vi "DrawArrowedLineOnImageARGB.vi"(4 "Thickness (Default: 1)":i32=1, 5 "Tip Length (Default 0.1)":dbl=0.1, 6 "ARGB Colour":T2={"Alpha"=255, "RGB"=0}, 7 "OpenCV Line Type (Default LINE_8)":T3=enum."LINE_8", 8 "error in (no error)":errorcluster, 9 "Pointed-to Point":T1, 10 "Start Point":T1, 11 "ARGB Image":refnum<data-value>) -> (0 "error out":errorcluster, 3 "ARGB Image (Duplicate)":refnum<data-value>)   [LabVIEW 2020, in "g_ar_toolkit.image.lvlib"]
uses:
  g_ar_toolkit.image.lvlib
  Line Type.ctl
  Image Point (Fixed).ctl
  ARGB Colour.ctl
  <vilib>/Utility/error.llb/Error Cluster From Error Code.vi
  c990ea83-8feb-41a3-987e-5529af170d73.vi
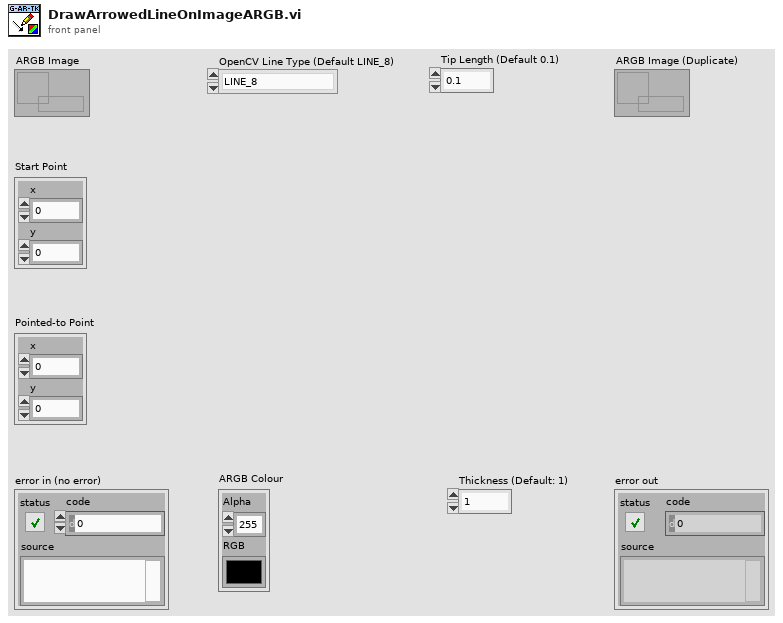
[diagram p1: front panel]
types:
  T1 = typedef "g_ar_toolkit.image.lvlib/Image Point (Fixed).ctl" = cluster{"x":i32, "y":i32}
  T2 = typedef "g_ar_toolkit.image.lvlib/ARGB Colour.ctl" = cluster{"Alpha":u8, "RGB":u32}
  T3 = typedef "g_ar_toolkit.image.lvlib/Line Type.ctl" = enum8{"FILLED", "LINE_4", "LINE_8", "LINE_AA"}
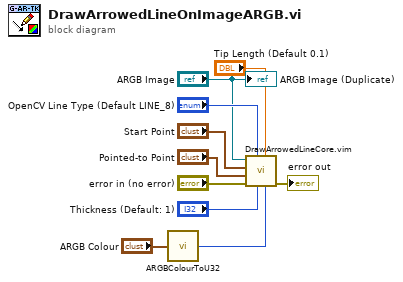
[diagram p0: block diagram]
diagram:
  n1 = call "ARGBColourToU32.vi"("ARGB Colour"="ARGB Colour") -> ("U32 Colour"=w4:u32)
  n2 = call "DrawArrowedLineCore.vim"("Colour"=w4, "Tip Length"="Tip Length (Default 0.1)", "Thickness"="Thickness (Default: 1)", "OpenCV Line Type"="OpenCV Line Type (Default LINE_8)", "error in (no error)"="error in (no error)", "Point B"="Pointed-to Point", "Point A"="Start Point", "Src"="ARGB Image") -> ("error out"=→"error out":errorcluster)  [unwired: 3 in]
  "ARGB Image (Duplicate)" <- "ARGB Image"
